vi "SM correction ver2.vi"(0 "V in x":dbl, 1 "nm in":dbl, 2 "V in y":dbl, 3 "V x initial":dbl, 4 "Volts/pixel":dbl, 5 "V y initial":dbl, 8 "Array":dbl[][](array[numeric])) -> (6 "V out x":dbl[](array[numeric]), 7 "V out y":dbl[](array[numeric]))   [LabVIEW 2010]
uses:
  <vilib>/measure/NI_MABase.lvlib
panel:
  out "V offset y":dbl
  out "V offset x":dbl
  # "deltax"
  # "nm"
  # "deltay"
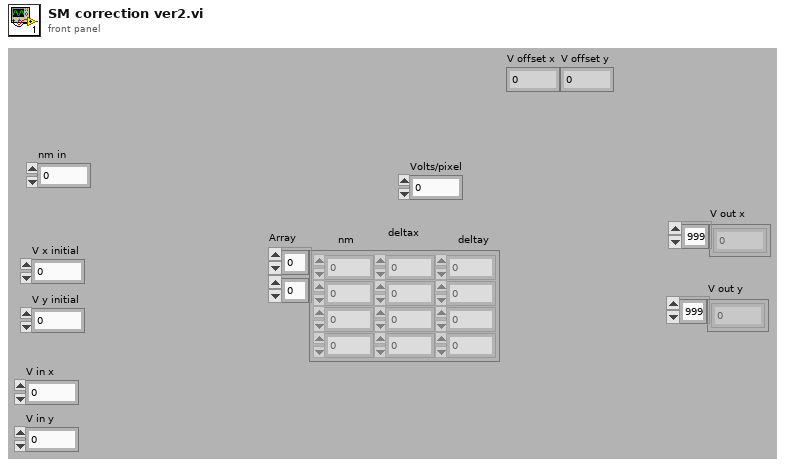
[diagram p1: front panel]
types:
  T1 = enum16{"Sine Wave", "Triangle Wave", "Square Wave", "Sawtooth Wave"}
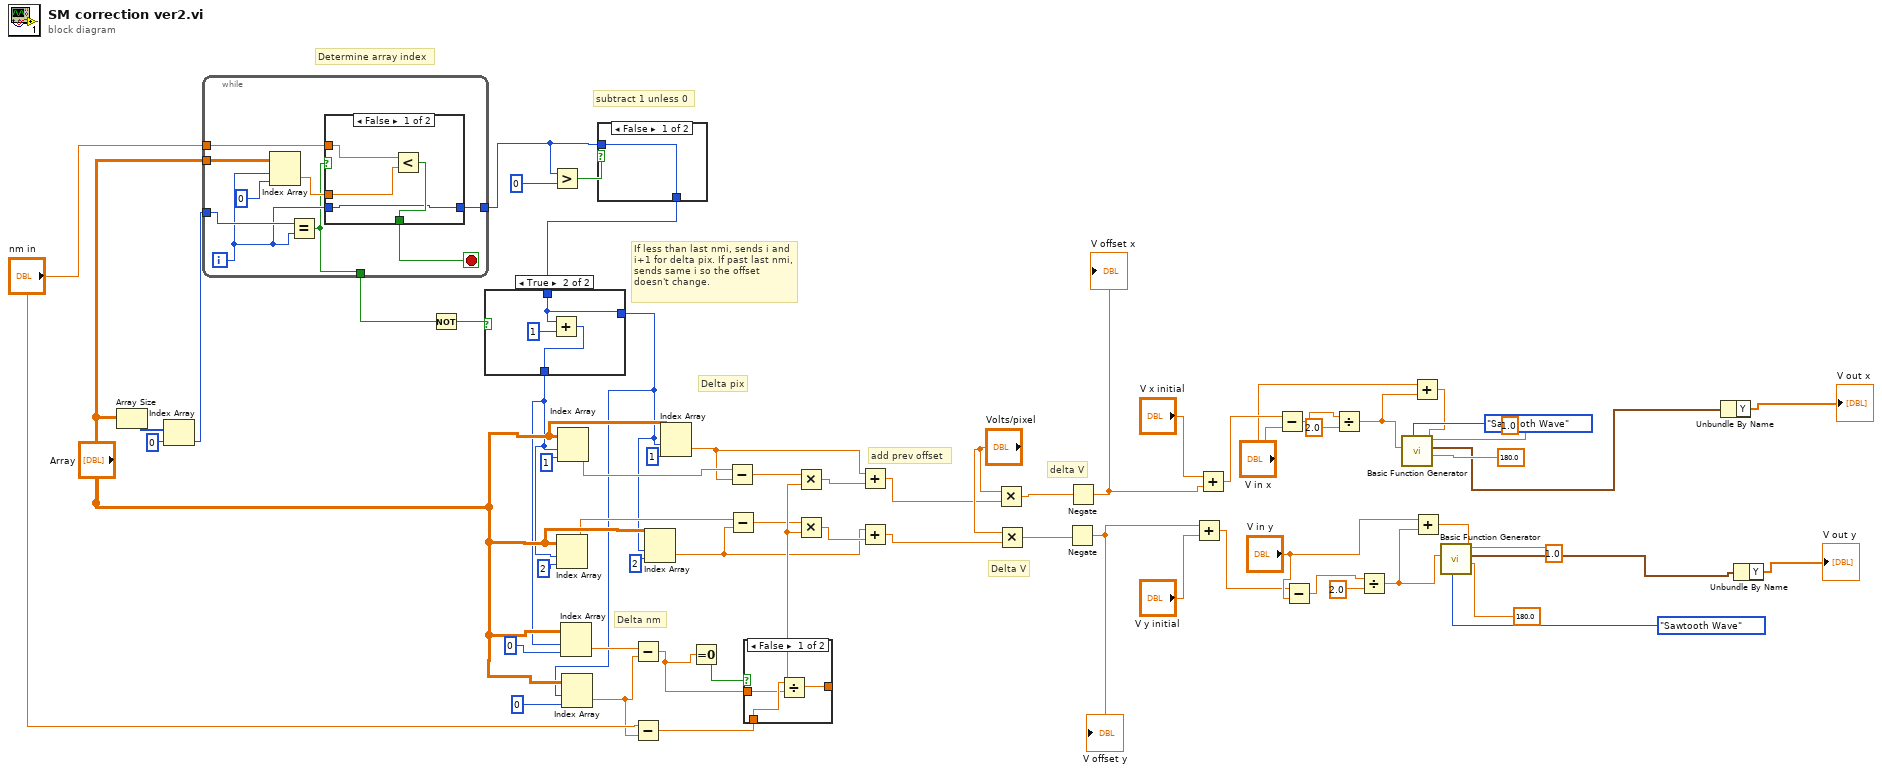
[diagram p0: block diagram]
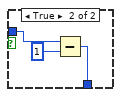
[diagram p4: hidden frame]
diagram:
  # "If less than last nmi, sends i and i+1 for delta pix. If past last nmi, sends same i so the offset doesn't change."
  # "delta V"
  # "add prev offset"
  # "subtract 1 unless 0"
  # "Determine array index"
  # "Delta nm"
  # "Delta V"
  # "Delta pix"
  n1 = Array Size(array="Array") -> (size(s)=w58:i32[])
  n2 = Index Array(array=w58, index=0) -> (element=w56:i32)
  n3 = while {
    tunnel: w56 -> [w72]
    tunnel: "nm in" -> [w69]
    tunnel: [w71] -> w52
    tunnel: "Array" -> [w67]
    tunnel: [w65] -> w7
    i -> [w66]
    stop <- w70 stop-if-true
    n4 = Index Array(array=w67, index (row)=w66, index (col)=0 ("disabled index (col)")) -> (element=w68:dbl)
    n5 = Equal?(x=w72, y=w66) -> (x = y?=w65:bool)
    n6 = case shown="False" w65 {
      selector: w65 -> [_ w78]
      tunnel: w66 -> [w74 w79]
      tunnel: [w74 w79] -> w71
      tunnel: [w75 w78] -> w70
      tunnel: w69 -> [w77 _]
      tunnel: w68 -> [w76 _]
      frame False {
        n7 = Less?(x=w77, y=w76) -> (x < y?=w75:bool)
      }
      frame True {
      }
    }
  }
  n8 = Not(x=w7) -> (.not. x?=w6:bool)
  n9 = Greater?(x=w52, y=0) -> (0:w53:bool)
  n10 = case shown="False" w53 {
    tunnel: w52 -> [w80 w83]
    tunnel: [w80 w81] -> w8
    frame False {
    }
    frame True {
      n11 = Subtract(x=w83, y=1) -> (x-y=w81:i32)
    }
  }
  n12 = case shown="True" w6 {
    tunnel: [w84 w86] -> w5
    tunnel: w8 -> [w84 w85]
    tunnel: [w84 w85] -> w4
    frame False {
    }
    frame True {
      n13 = Add(x=w85, y=1) -> (x+y=w86:i32)
    }
  }
  n14 = Index Array(array="Array", index (row)=w5, index (col)=2 ("index")) -> (element=w46:dbl)
  n15 = Index Array(array="Array", index (row)=w5, index (col)=1 ("index")) -> (element=w47:dbl)
  n16 = Index Array(array="Array", index (row)=w5, index (col)=0 ("index")) -> (element=w63:dbl)
  n17 = Index Array(array="Array", index (row)=w4, index (col)=0 ("index")) -> (element=w1:dbl)
  n18 = Subtract(x=w63, y=w1) -> (x-y=w2:dbl)
  n19 = Subtract(x="nm in", y=w1) -> (x-y=w51:dbl)
  n20 = Index Array(array="Array", index (row)=w4, index (col)=2) -> (element=w40:dbl)
  n21 = Index Array(array="Array", index (row)=w4, index (col)=1) -> (element=w39:dbl)
  n22 = Equal To 0?(x=w2) -> (x = 0?=w3:bool)
  n23 = Subtract(x=w47, y=w39) -> (x-y=w44:dbl)
  n24 = Subtract(x=w46, y=w40) -> (x-y=w43:dbl)
  n25 = case shown="False" w3 {
    tunnel: w51 -> [w90 _]
    tunnel: w2 -> [w89 w91]
    tunnel: [w88 w91] -> w45
    frame False {
      n26 = Divide(x=w90, y=w89) -> (x/y=w88:dbl)
    }
    frame True {
      # "Frac range"
    }
  }
  n27 = Multiply(x=w44, y=w45) -> (x*y=w42:dbl)
  n28 = Multiply(x=w43, y=w45) -> (x*y=w41:dbl)
  n29 = Add(x=w39, y=w42) -> (x+y=w38:dbl)
  n30 = Add(x=w40, y=w41) -> (x+y=w37:dbl)
  n31 = Multiply(x="Volts/pixel", y=w38) -> (x*y=w33:dbl)
  n32 = Multiply(x="Volts/pixel", y=w37) -> (x*y=w29:dbl)
  n33 = Negate(x=w29) -> (-x=w27:dbl)
  "V offset y" <- w27
  n34 = Negate(x=w33) -> (-x=w28:dbl)
  "V offset x" <- w28
  n35 = Add(x=w27, y="V y initial") -> (x+y=w13:dbl)
  n36 = Add(x="V x initial", y=w28) -> (x+y=w26:dbl)
  n37 = Subtract(x=w26, y="V in x") -> (x-y=w24:dbl)
  n38 = Subtract(x=w13, y="V in y") -> (x-y=w18:dbl)
  n39 = Divide(x=w24, y=2.0) -> (x/y=w21:dbl)
  n40 = Divide(x=w18, y=2.0) -> (x/y=w16:dbl)
  n41 = Add(x="V in x", y=w21) -> (x+y=w20:dbl)
  n42 = call <vilib>:"Basic Function Generator.vi"("offset"=w20, "signal type"=T1."Sawtooth Wave", "phase"=180.0, "amplitude"=w21, "frequency"=1.0) -> ("signal out"=w12:waveform(dbl))  [unwired: 4 in, 2 out]
  n43 = Add(x="V in y", y=w16) -> (x+y=w15:dbl)
  n44 = call <vilib>:"Basic Function Generator.vi"("offset"=w15, "signal type"=T1."Sawtooth Wave", "phase"=180.0, "amplitude"=w16, "frequency"=1.0) -> ("signal out"=w11:waveform(dbl))  [unwired: 4 in, 2 out]
  n45 = Unbundle By Name(w12) -> ("Y"=→"V out x":dbl[])
  n46 = Unbundle By Name(w11) -> ("Y"=→"V out y":dbl[])
